vi "UpdateClassApperance.vi"(0 "ClassRefIn":refnum<vi>, 2 "MessageClass(False)":bool, 5 "error in (no error)":errorcluster) -> (14 "ClassRefOut":refnum<vi>, 19 "error out":errorcluster)   [LabVIEW 2012, in "ClassWriter.lvclass"]
uses:
  <resource>/Framework/Providers/Open_GDS/ClassProviders/Provider_BaseClassInterface/ClassWriter_class/ClassWriter.lvclass
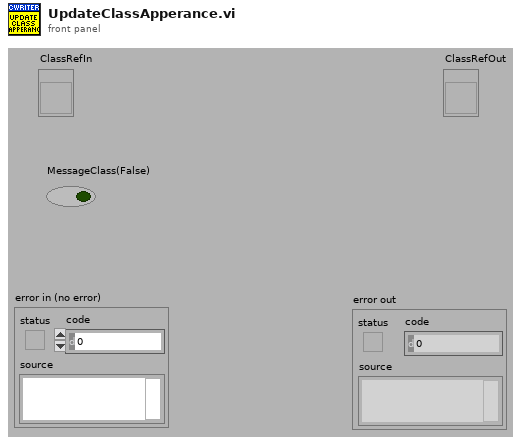
[diagram p1: front panel]
types:
  T1 = typedef "GOOP_WireConfigurationType.ctl" = cluster{"Edge thickness":i32, "Edge color":u32, "Center thickness":i32, "Center pattern":T2, "CenterColor1":u32, "CenterColor2":u32, "Tunnels and terminals colors":u32}
  T2 = typedef "GOOP_WirePattern.ctl" = enum16{"Solid", "Large dash", "Small dash"}
  T3 = cluster{"Foreground Color":u32, "Background Color":u32, "Fill Pattern":cluster{"Row 0":u8, "Row 1":u8, "Row 2":u8, "Row 3":u8, "Row 4":u8, "Row 5":u8, "Row 6":u8, "Row 7":u8}, "Width":i16, "Mode":enum16{"Copy", "Or", "Exclusive Or", "Bit Clear", "Not Copy", "Not Or", "Nor Exclusive Or", "Not Bit Clear"}, "Style":enum32{"Solid", "Dash", "Dot", "Dash Dot", "Dash Dot Dot"}, "Fill Rule":enum32{"Even Odd", "Winding"}, "End Caps":enum32{"Default", "Flat"}}[]
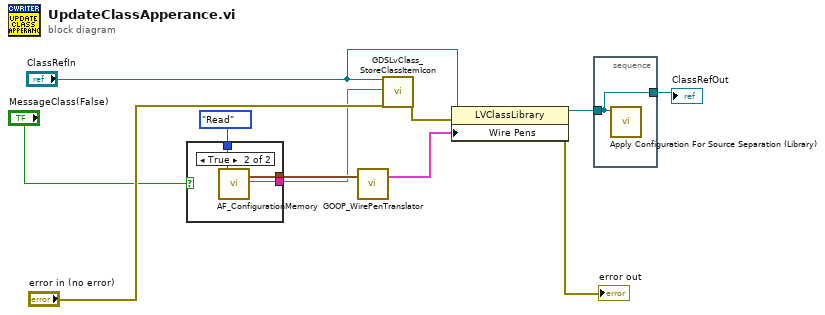
[diagram p0: block diagram]
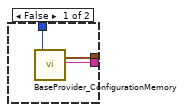
[diagram p2: hidden frame]
diagram:
  n1 = case shown="True" "MessageClass(False)" {
    tunnel: [w14 w16] -> w11
    tunnel: [w13 w15] -> w7
    tunnel: enum16{"Read", "Load", "Save", "Set"}."Read" ("Action") -> [w12 w17]
    frame False {
      n2 = call <resource>:"BaseProvider_ConfigurationMemory.vi"("Action"=w12) -> ("WireConfigurationOut"=w14:T1, "IconOut"=w13:string)  [unwired: 12 in, 5 out]
    }
    frame True {
      n3 = call <resource>:"AF_ConfigurationMemory.vi"("Action"=w17) -> ("AF_MessaageWireConfigurationOut"=w16:T1, "IconOut"=w15:string)  [unwired: 15 in, 2 out]
    }
  }
  n4 = call <resource>:"GOOP_WirePenTranslator.vi"("WireConfigurationIn"=w11) -> ("WirePensOut"=w10:T3)  [unwired: 17 in, 1 out]
  n5 = call <resource>:"GDSLvClass_StoreClassItemIcon.vi"("Library Refnum"="ClassRefIn", "ClassItemIconName"=w7, "error in (no error)"="error in (no error)") -> ("error out"=w9:errorcluster)  [unwired: 15 in, 1 out]
  n6 = property class="LVClassLibrary"(reference="ClassRefIn", error in=w9, "Wire Pens"=w10) -> (reference out=w2:refnum<vi>, error out=→"error out":errorcluster)
  n7 = stacked-sequence {
    tunnel: w2 -> [w18]
    tunnel: [w18] -> w1
    frame #0 {
      n8 = call <vilib>:"Apply Configuration For Source Separation (Library).vi"("Library in"=w18) -> ()  [unwired: 9 in, 2 out]
    }
  }
  "ClassRefOut" <- w1
